vi "Handle Error.vi"(8 "error in (no error)":errorcluster, 11 "Console in":refnum<class "Console.lvclass">) -> (0 "error out":errorcluster, 2 "stop actor?":bool=TRUE, 3 "Console out":refnum<class "Console.lvclass">)   [LabVIEW 2015, in "EditPanel API.lvlib" / "Console.lvclass"]
doc: "(<B>Filename</B>: Actor Framework.lvlib:Actor.lvclass:Handle Error.vi)\n\nDefines how the actor handles an error that occurred while processing a message. By default, this method does nothing except stop the actor."
uses:
  Console.lvclass
  Console Reply/Console Reply Error Report/Console Reply Error Report.lvclass
  Type Definition/Console_Q Data Type.ctl
  Console Reply/Console Reply/Console Reply.lvclass
  Panel Control_Interface/Panel_interface/Panel Controller Interface.lvclass
  Console.lvclass/Console.ctl
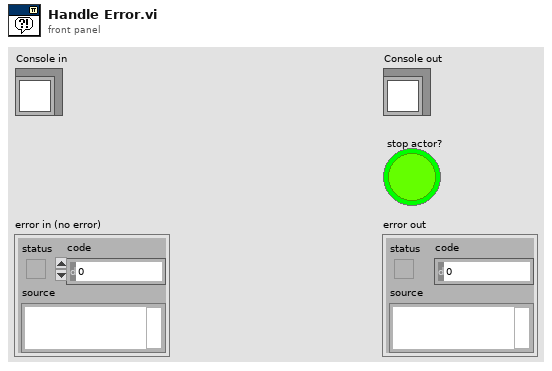
[diagram p1: front panel]
types:
  T1 = typedef "EditPanel API.lvlib/Console.lvclass/Console_Q Data Type.ctl" = cluster{"Console Reply":refnum<class "Console Reply.lvclass">, "Panel":refnum<class "Panel Controller Interface.lvclass">}
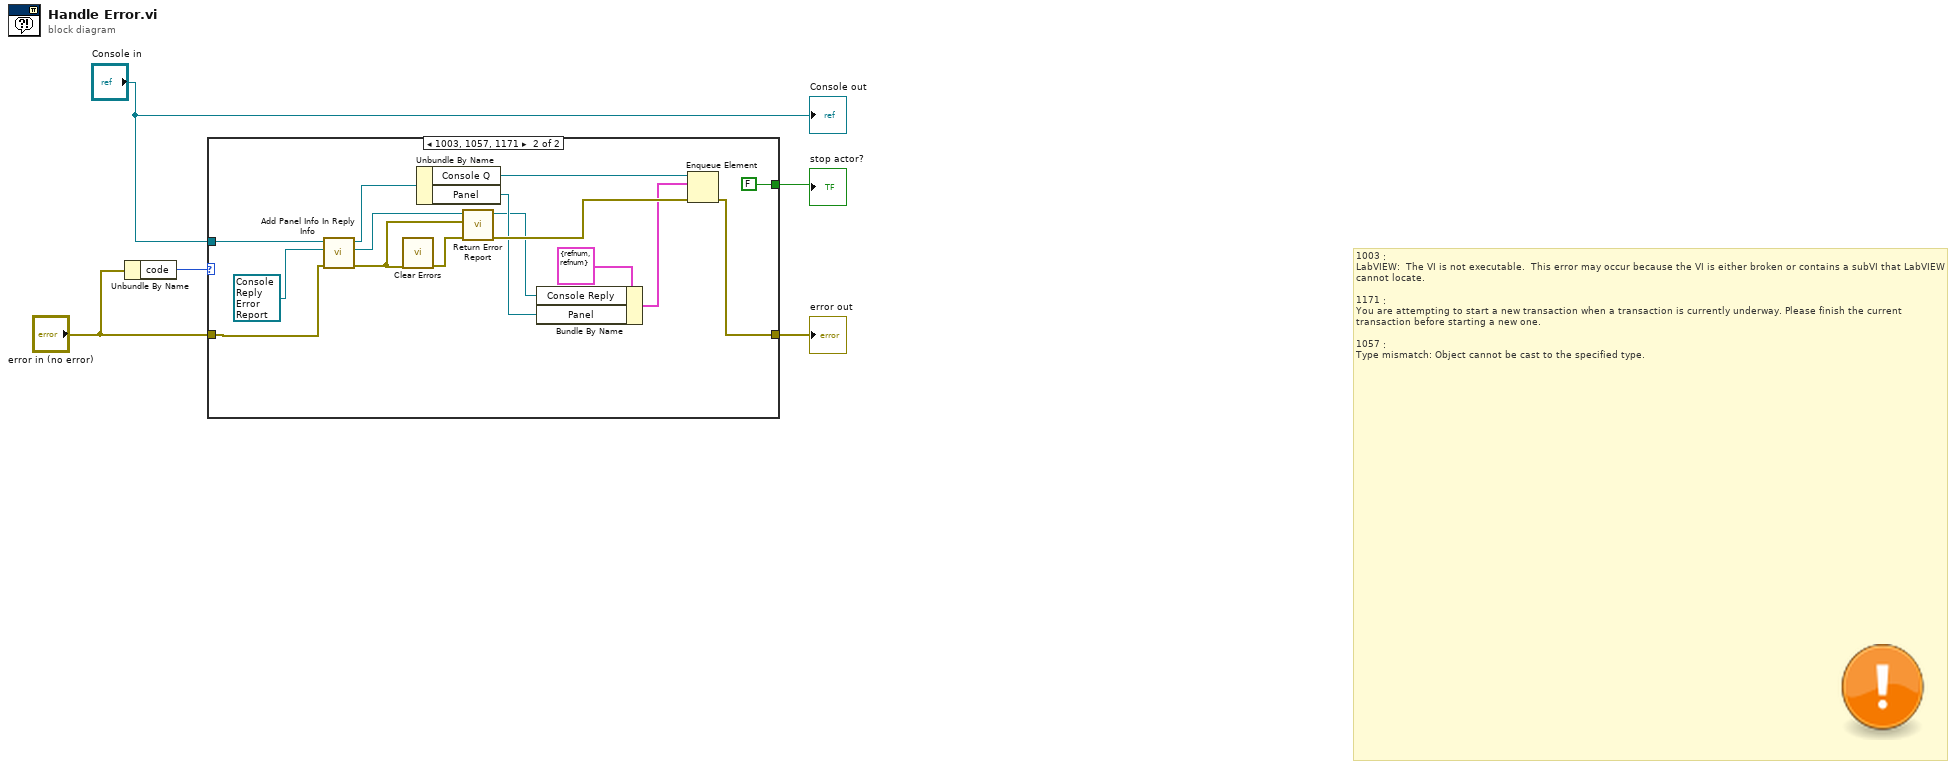
[diagram p0: block diagram]
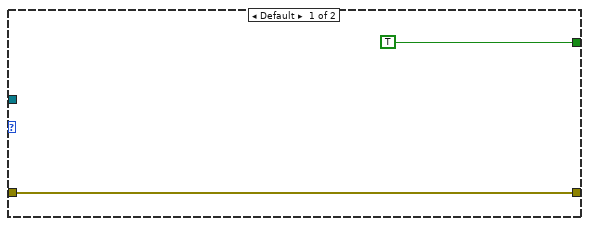
[diagram p2: hidden frame]
diagram:
  # "1003：\nLabVIEW:  The VI is not executable.  This error may occur because the VI is either broken or contains a subVI that LabVIEW cannot locate.\n\n1171：\nYou are attempting to start a new transaction when a transaction is currently underway. Please finish the current transaction before starting a new one.\n\n1057：\nType mismatch: Object cannot be cast to the specified type."
  n1 = Unbundle By Name("error in (no error)") -> ("code"=w5:i32)
  n2 = case shown="1003, 1057, 1171" w5 {
    tunnel: "Console in" -> [_ w18]
    tunnel: "error in (no error)" -> [w7 w16]
    tunnel: [w7 w19] -> w3
    tunnel: [TRUE FALSE] -> w2
    frame Default {
    }
    frame 1003, 1057, 1171 {
      n3 = call "Add Panel Info In Reply Info.vi"("error in (no error)"=w16, "Reply"=refnum<class "Console Reply Error Report.lvclass"> refnum ("Console Error(Console2API) in"), "Console in"=w18) -> ("error out"=w13:errorcluster, "Console2API Q out"=w15:refnum<class "Console Reply Error Report.lvclass">, "Console out"=w14:refnum<class "Console.lvclass">)  [unwired: 6 in]
      n4 = call <vilib>:"Clear Errors.vi"("error in (no error)"=w13) -> ("error out"=w12:errorcluster)  [unwired: 5 in, 1 out]
      n5 = Unbundle By Name(w14) -> ("Console Q"=w22:refnum<queue>, "Panel"=w10:refnum<class "Panel Controller Interface.lvclass">)
      n6 = call "Return Error Report.vi"("error in (no error)"=w12, "error Source(No Error)"=w13, "Console Error(Console2API) in"=w15) -> ("error out"=w20:errorcluster, "Console Error(Console2API) out"=w9:refnum<class "Console Reply Error Report.lvclass">)  [unwired: 7 in]
      n7 = Bundle By Name(cluster=T1 {"Console Reply"=refnum, "Panel"=refnum} ("element"), "Console Reply"=w9, "Panel"=w10) -> (w8:T1)
      n8 = Enqueue Element(queue=w22, element=w8, error in (no error)=w20) -> (error out=w19:errorcluster)  [unwired: 1 in, 2 out]
    }
  }
  "error out" <- w3
  "stop actor?" <- w2
  "Console out" <- "Console in"
